vi "MQTT_SSL_Connect.vi"(5 "Connect Meta":T6={"Retain"=FALSE, "DUP"=FALSE, "Keep Alive (sec)"=60, "QoS"=enum."At most once"}, 6 "Client ID":string="LabVIEW_MQTT_Client", 7 "Connect Flags":T4, 8 "error in (no error)":errorcluster, 9 "Will Info":T9={"Will message"="Last Will", "Will Topic"="Will Topic"}, 10 "cert path":T1={"client cert file"=path "", "client key file"=path ""}, 11 "MQTT Broker":cluster{"address (IP)":string, "port":u16}={"address (IP)"="broker.mqttdashboard.com", "port"=1883}) -> (0 "error out":errorcluster, 2 "Connection Status":T10=enum."Connection refused: not authorized", 3 "SSL_Connection":T2)   [LabVIEW 2018, in "AWS_IoT.lvlib"]
uses:
  AWS_IoT.lvlib
  Controls/Connection_Return_Codes.ctl
  Controls/Will_Info.ctl
  Controls/ConnectMeta.ctl
  Controls/Retain_Flag.ctl
  Controls/DUP_Flag.ctl
  Controls/QoS.ctl
  Controls/Connect_Flags.ctl
  Controls/SSL_login.ctl
  Controls/SSL_Connection.ctl
  Controls/certs.ctl
  Controls/MessageType.ctl
  Controls/Conn_Stat_FGV_Cmds.ctl
panel:
  in  "SSL_Connection":T2
  in  "login":T3={"server IP"="", "server port"=0, "local port (0 = auto)"=0, "timeout ms (1000)"=1000}
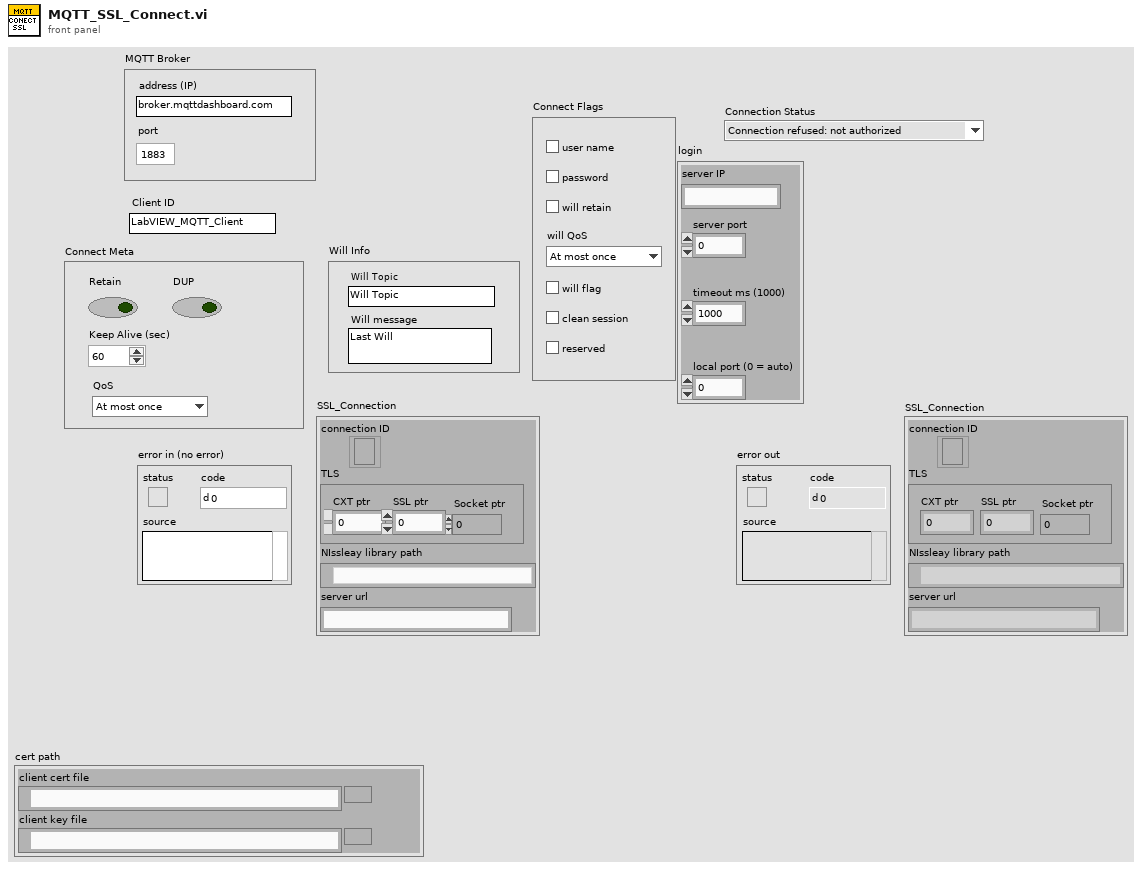
[diagram p1: front panel]
types:
  T1 = typedef "AWS_IoT.lvlib/certs.ctl" = cluster{"client cert file":path, "client key file":path}
  T2 = typedef "AWS_IoT.lvlib/SSL_Connection.ctl" = cluster{"connection ID":refnum<k5>, "TLS":cluster{"CXT ptr":i32, "SSL ptr":i32, "Socket ptr":i32}, "NIssleay library path":path, "server url":string}
  T3 = typedef "AWS_IoT.lvlib/SSL_login.ctl" = cluster{"server IP":string, "server port":u16, "local port (0 = auto)":u16, "timeout ms (1000)":i32}
  T4 = typedef "AWS_IoT.lvlib/Connect_Flags.ctl" = cluster{"user name":bool, "password":bool, "will retain":bool, "will flag":bool, "clean session":bool, "reserved":bool, "will QoS":T5}
  T5 = typedef "AWS_IoT.lvlib/QoS.ctl" = enum8{"At most once", "At least once", "Exactly once", "Reserved"}
  T6 = typedef "AWS_IoT.lvlib/ConnectMeta.ctl" = cluster{"Retain":T7, "DUP":T8, "Keep Alive (sec)":u16, "QoS":T5}
  T7 = typedef "AWS_IoT.lvlib/Retain_Flag.ctl" = bool
  T8 = typedef "AWS_IoT.lvlib/DUP_Flag.ctl" = bool
  T9 = typedef "AWS_IoT.lvlib/Will_Info.ctl" = cluster{"Will message":string, "Will Topic":string}
  T10 = typedef "AWS_IoT.lvlib/Connection_Return_Codes.ctl" = enum16{"Connection accepted", "Connection refused: unacceptable protocol version", "Connection refused: identifier rejected", "Connection refused: Server unavailable", "Connection refused: bad user name or password", "Connection refused: not authorized"}
  T11 = typedef "AWS_IoT.lvlib/Conn_Stat_FGV_Cmds.ctl" = enum16{"Get", "Set"}
  T12 = typedef "AWS_IoT.lvlib/MessageType.ctl" = enum32{"Reserved", "CONNECT", "CONNACK", "PUBLISH", "PUBACK", "PUBREC", "PUBREL", "PUBCOMP", "SUBSCRIBE", "SUBACK", "UNSUBSCRIBE", "UNSUBACK", "PINGREQ", "PINGRESP", "DISCONNECT", "Reserved2"}
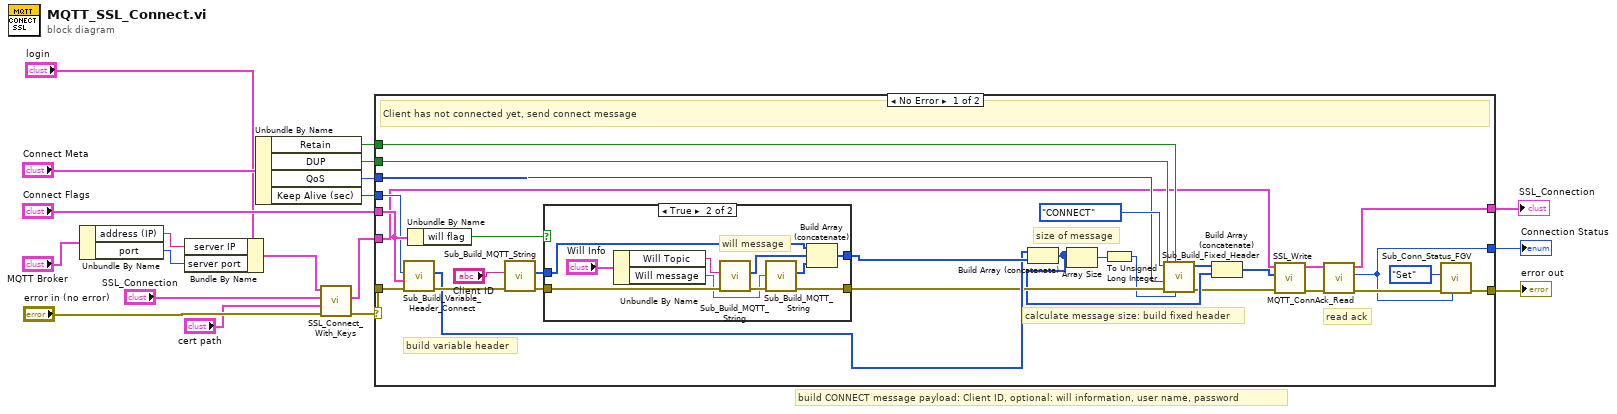
[diagram p0: block diagram]
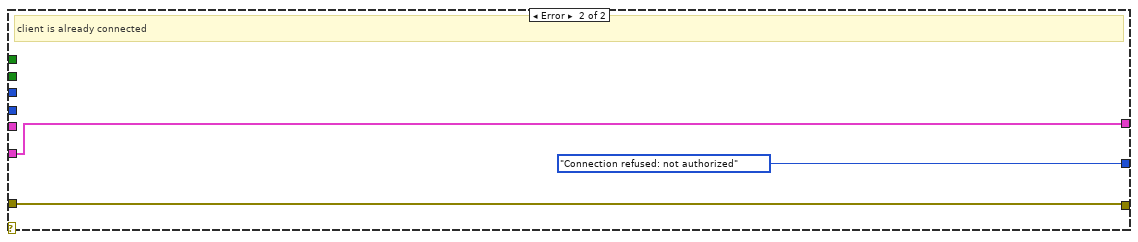
[diagram p3: hidden frame]
diagram:
  # "build CONNECT message payload: Client ID, optional: will information, user name, password"
  n1 = Unbundle By Name("MQTT Broker") -> ("address (IP)"=w8:string, "port"=w7:u16)
  n2 = Bundle By Name(cluster="login", "server IP"=w8, "server port"=w7) -> (w11:T3)
  n3 = Unbundle By Name("Connect Meta") -> ("Retain"=w15:T7, "DUP"=w16:T8, "QoS"=w17:T5, "Keep Alive (sec)"=w18:u16)
  n4 = call "SSL_Connect_With_Keys.vi"("error in (no error)"="error in (no error)", "cert path"="cert path", "SSL_Connection"="SSL_Connection", "login"=w11) -> ("error out"=w4:errorcluster, "SSL_Connection"=w1:T2)  [unwired: 6 in]
  n5 = case shown="No Error" w4 {
    tunnel: "Connect Flags" -> [w43 _]
    tunnel: w15 -> [w35 _]
    tunnel: w16 -> [w34 _]
    tunnel: w17 -> [w33 _]
    tunnel: w18 -> [w32 _]
    tunnel: w4 -> [w28 w63]
    tunnel: [w24 w63] -> w19
    tunnel: [w27 w61] -> w5
    tunnel: [w23 Connection_Return_Codes."Connection refused: not authorized" ("Connection Status")] -> w3
    tunnel: w1 -> [w21 w61]
    frame No Error {
      # "read ack"
      # "calculate message size: build fixed header"
      # "build variable header"
      # "size of message"
      # "Client has not connected yet, send connect message"
      n6 = call "Sub_Build_Variable_Header_Connect.vi"("error in (no error)"=w28, "Connect Flags"=w43, "Keep Alive (sec)"=w32) -> ("error out"=w47:errorcluster, "Variable Header"=w41:u8[])  [unwired: 7 in]
      n7 = Unbundle By Name(w43) -> ("will flag"=w42:bool)
      n8 = call "Sub_Build_MQTT_String.vi"("error in (no error)"=w47, "String to be encoded"="Client ID") -> ("error out"=w44:errorcluster, "UTF8 Byte Array"=w46:u8[])  [unwired: 8 in]
      n9 = case shown="True" w42 {
        tunnel: w46 -> [w50 w58]
        tunnel: [w50 w59] -> w45
        tunnel: w44 -> [w49 w57]
        tunnel: [w49 w54] -> w40
        frame False {
        }
        frame True {
          # "will message"
          n10 = Unbundle By Name("Will Info") -> ("Will Topic"=w52:string, "Will message"=w51:string)
          n11 = call "Sub_Build_MQTT_String.vi"("error in (no error)"=w57, "String to be encoded"=w52) -> ("error out"=w56:errorcluster, "UTF8 Byte Array"=w55:u8[])  [unwired: 8 in]
          n12 = call "Sub_Build_MQTT_String.vi"("error in (no error)"=w56, "String to be encoded"=w51) -> ("error out"=w54:errorcluster, "UTF8 Byte Array"=w60:u8[])  [unwired: 8 in]
          n13 = Build Array (concatenate)(w58, w55, w60) -> (w59:u8[])
        }
      }
      n14 = Build Array (concatenate)(w41, w45) -> (w39:u8[])
      n15 = Array Size(array=w39) -> (size(s)=w37:i32)
      n16 = To Unsigned Long Integer(number=w37) -> (unsigned 32bit integer=w36:u32)
      n17 = call "Sub_Build_Fixed_Header.vi"("Remaining Length"=w36, "Retain"=w35, "error in (no error)"=w40, "QoS"=w33, "DUP"=w34, "MessageType"=MessageType."CONNECT") -> ("error out"=w30:errorcluster, "Fixed Header"=w38:u8[])  [unwired: 4 in]
      n18 = Build Array (concatenate)(w38, w39) -> (w22:u8[])
      n19 = call "SSL_Write.vi"("error in (no error)"=w30, "data in"=w22, "SSL_Connection"=w21) -> ("error out"=w29:errorcluster, "SSL_Connection"=w20:T2)  [unwired: 7 in]
      n20 = call "MQTT_ConnAck_Read.vi"("error in (no error)"=w29, "SSL_Connection"=w20) -> ("error out"=w26:errorcluster, "Connection Status"=w23:T10, "SSL_Connection"=w27:T2)  [unwired: 5 in, 2 out]
      n21 = call "Sub_Conn_Status_FGV.vi"("Connection Status in"=w23, "error in"=w26, "Command"=Conn_Stat_FGV_Cmds."Set") -> ("error out"=w24:errorcluster)  [unwired: 7 in, 1 out]
    }
    frame Error {
      # "client is already connected"
    }
  }
  "error out" <- w19
  "Connection Status" <- w3
  "SSL_Connection" <- w5
